vi "Plot Load maker V2 - scaleread grid colors.vi"(8 "error in (no error)":errorcluster, 10 "Scale reference":refnum<vi>, 11 "Meta LUT":refnum<data-value>) -> (0 "error out":errorcluster, 1 "Scale LUT meta":T1, 2 "Scale reference":refnum<vi>, 3 "Meta LUT":refnum<data-value>)   [LabVIEW 2021, in "RocketPlot.lvlib"]
uses:
  RocketPlot.lvlib
  TypeDefs/Plot scale meta JSON.ctl
  TypeDefs/Plot axis.ctl
  TypeDefs/Plot scale meta state.ctl
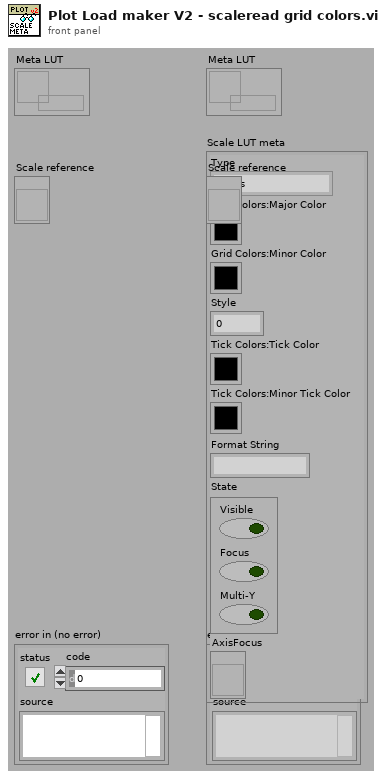
[diagram p1: front panel]
types:
  T1 = typedef "RocketPlot.lvlib/Plot scale meta JSON.ctl" = cluster{"Type":T2, "Grid Colors:Major Color":u32, "Grid Colors:Minor Color":u32, "Style":u8, "Tick Colors:Tick Color":u32, "Tick Colors:Minor Tick Color":u32, "Format String":string, "State":T3, "AxisFocus":refnum<vi>}
  T2 = typedef "RocketPlot.lvlib/Plot axis.ctl" = enum16{"x axis", "left axis", "right axis"}
  T3 = typedef "RocketPlot.lvlib/Plot scale meta state.ctl" = cluster{"Visible":bool, "Focus":bool, "Multi-Y":bool}
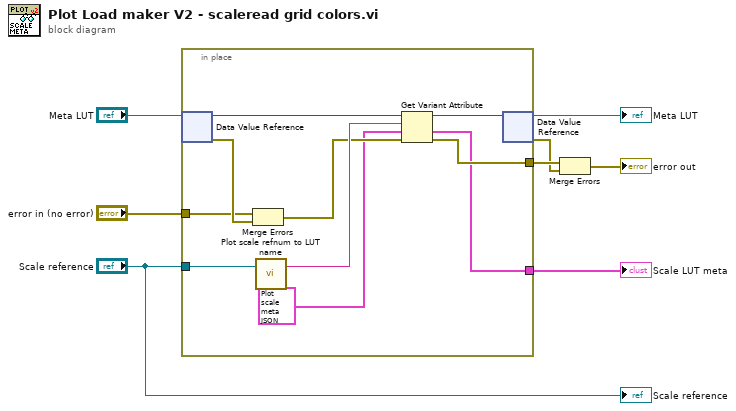
[diagram p0: block diagram]
diagram:
  n1 = in-place {
    in-place-border: "Scale reference" -> [w18]
    in-place-border: "error in (no error)" -> [w13]
    in-place-border: [w11] -> w5
    in-place-border: [w9] -> w6
    n2 = in-place-dvr #1("Meta LUT") -> (w16:variant, w14:errorcluster)
    n3 = Merge Errors(w13, w14) -> (w12:errorcluster)
    n4 = call "Plot scale refnum to LUT name.vi"("Scale reference"=w18) -> ("scale reference variant lookup name"=w17:string)  [unwired: 2 in]
    n5 = Get Variant Attribute(Variant=w16, name=w17, default value (empty Variant)=T1 {"Type"=enum."x axis", "Grid Colors:Major Color"=0, "Grid Colors:Minor Color"=0, "Style"=0, "Tick Colors:Tick Color"=0, "Tick Colors:Minor Tick Color"=0, "Format String"="", "State"={"Visible"=FALSE, "Focus"=FALSE, "Multi-Y"=FALSE}, "AxisFocus"=refnum} ("Meta"), error in=w12) -> (duplicate Variant=w15:variant, value=w9:T1, error out=w11:errorcluster)  [unwired: 1 out]
    n6 = in-place-dvr #1(w15) -> (→"Meta LUT":refnum<data-value>, w4:errorcluster)
  }
  "Scale LUT meta" <- w6
  n7 = Merge Errors(w5, w4) -> (→"error out":errorcluster)
  "Scale reference" <- "Scale reference"
